vi "Write datatype.vi"(8 "error in (no error)":errorcluster, 10 "datatype":T1, 11 "JSON Datatype in":refnum<class "JSON Datatype.lvclass">=refnum) -> (0 "error out":errorcluster, 3 "JSON Datatype out":refnum<class "JSON Datatype.lvclass">)   [LabVIEW 2017]
uses:
  JSON Datatype.lvclass
  JSON Types.ctl
  LVJSON.lvlib
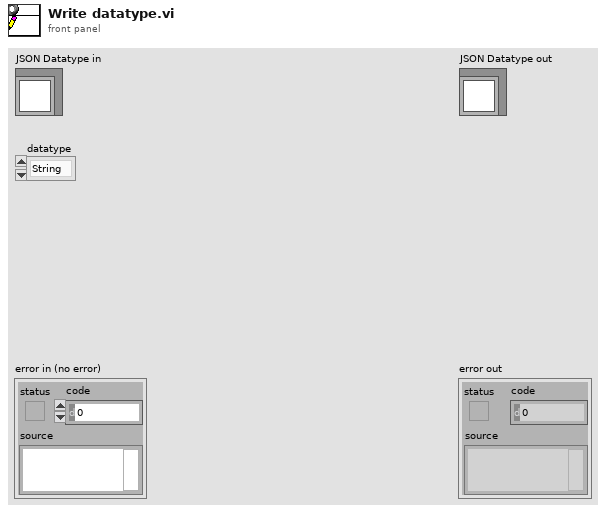
[diagram p1: front panel]
types:
  T1 = typedef "LVJSON.lvlib/JSON Types.ctl" = enum16{"String", "Numeric", "Boolean", "NULL", "Object", "1D Array", "Unknown"}
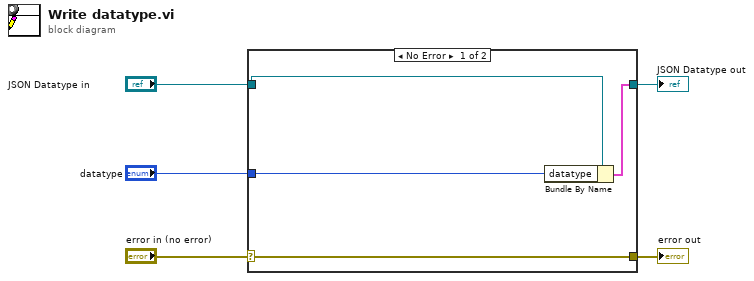
[diagram p0: block diagram]
diagram:
  n1 = case shown="No Error" "error in (no error)" {
    selector: "error in (no error)" -> [w9 w10]
    tunnel: [w9 w10] -> w4
    tunnel: [w7 w11] -> w2
    tunnel: "JSON Datatype in" -> [w8 w11]
    tunnel: "datatype" -> [w6 _]
    frame No Error {
      n2 = Bundle By Name(cluster=w8, "datatype"=w6) -> (w7:cluster{})
    }
    frame Error {
    }
  }
  "error out" <- w4
  "JSON Datatype out" <- w2
